vi "_Parse Session Content.vi"(11 "Text":string) -> (2 "Section":string[](array[string]), 3 "SectionContent":string[](array[string]))   [LabVIEW 2017, in "LabVIEW-Config.lvlib" / "LabVIEW-Config.lvclass"]
uses:
  LabVIEW-Config.lvclass
  LineToken.ctl
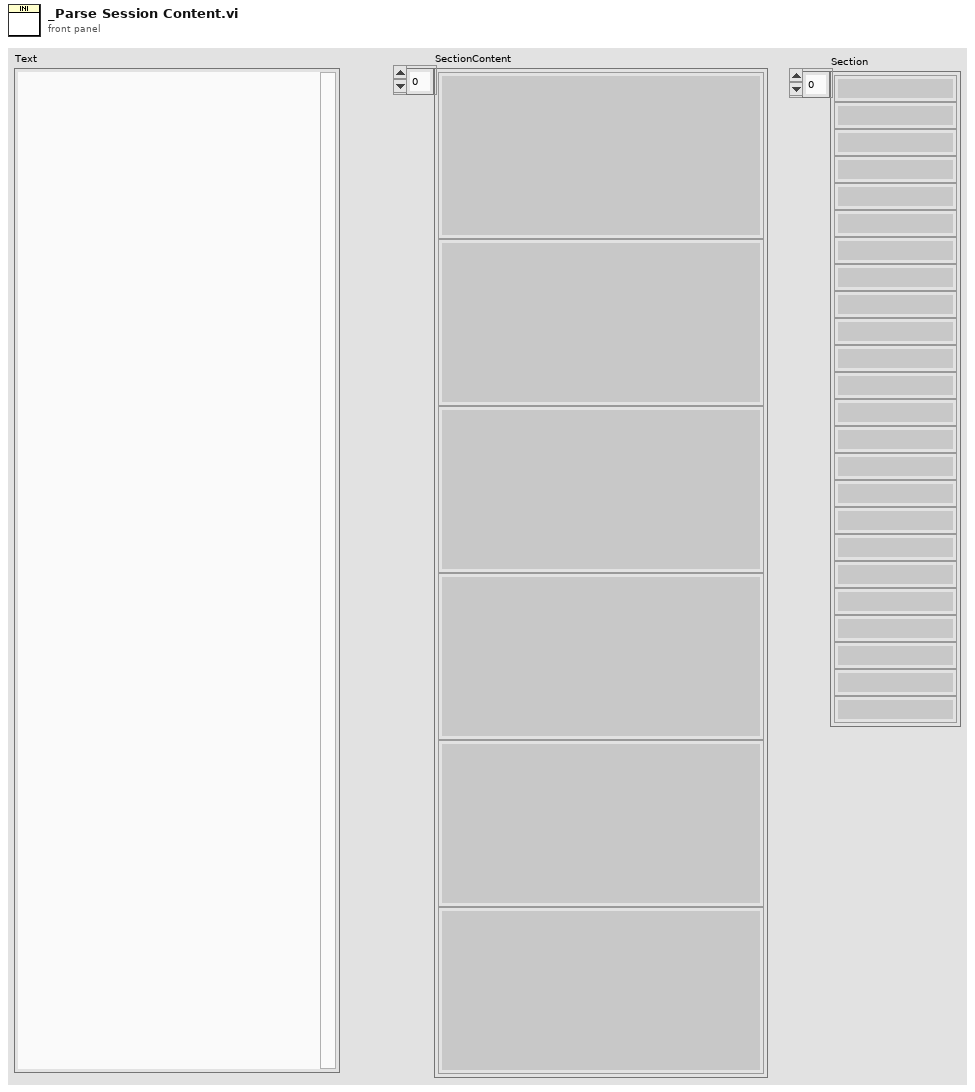
[diagram p1: front panel]
types:
  T1 = typedef "LabVIEW-Config.lvlib/LabVIEW-Config.lvclass/LineToken.ctl" = enum8{"comment", "section", "key", "more"}
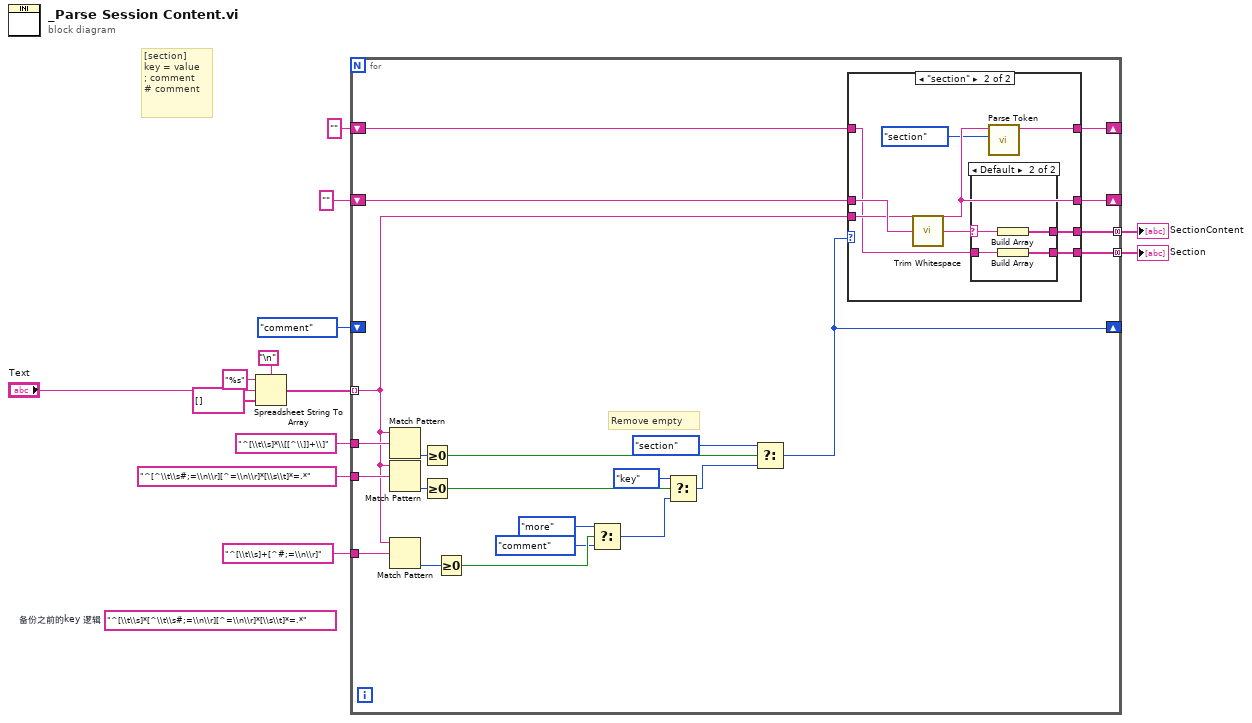
[diagram p0: block diagram]
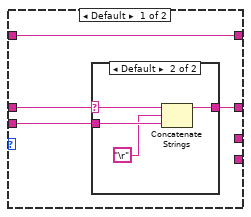
[diagram p2: hidden frame]
diagram:
  (unwired) "^[\\t\\s]*[^\\t\\s#;=\\n\\r][^=\\n\\r]*[\\s\\t]*=.*"  # 备份之前的key 逻辑
  # "[section]\nkey = value\n; comment\n# comment"
  n1 = Spreadsheet String To Array(delimiter (Tab)="\n" ("Line Feed Constant"), format string="%s", spreadsheet string="Text", array type (2D Dbl)=string[] []) -> (array=w11:string[])
  n2 = for {
    tunnel: w11 -> [w17] mode=indexing
    tunnel: "^[\\t\\s]*\\[[^\\]]+\\]" ("regular expression") -> [w36]
    tunnel: "^[^\\t\\s#;=\\n\\r][^=\\n\\r]*[\\s\\t]*=.*" ("regular expression") -> [w33]
    tunnel: "^[\\t\\s]+[^#;=\\n\\r]" ("regular expression") -> [w26]
    shift-right: [w21] -> _
    shift-left: LineToken."comment" ("Token") -> [_]
    shift-right: [w18] -> _
    shift-left: "" ("regular expression") -> [w20]
    tunnel: [w19] -> w3 mode=concatenating
    shift-right: [w16] -> _
    shift-left: "" ("Name") -> [w15]
    tunnel: [w14] -> w1 mode=concatenating
    # "Remove empty"
    n3 = Match Pattern(string=w17, regular expression=w36) -> (offset past match=w35:i32)  [unwired: 1 in, 3 out]
    n4 = Match Pattern(string=w17, regular expression=w33) -> (offset past match=w34:i32)  [unwired: 1 in, 3 out]
    n5 = Match Pattern(string=w17, regular expression=w26) -> (offset past match=w27:i32)  [unwired: 1 in, 3 out]
    n6 = Greater Or Equal To 0?(x=w35) -> (x >= 0?=w32:bool)
    n7 = Greater Or Equal To 0?(x=w34) -> (x >= 0?=w28:bool)
    n8 = Greater Or Equal To 0?(x=w27) -> (x >= 0?=w25:bool)
    n9 = Select(t=LineToken."more" ("Token"), s=w25, f=LineToken."comment" ("Token")) -> (s? t:f=w22:T1)
    n10 = Select(t=LineToken."key" ("Token"), s=w28, f=w22) -> (s? t:f=w29:T1)
    n11 = Select(t=LineToken."section" ("Token"), s=w32, f=w29) -> (s? t:f=w21:T1)
    n12 = case shown="\"section\"" w21 {
      tunnel: w20 -> [w40 w53]
      tunnel: [_ w52] -> w19
      tunnel: [w39 w50] -> w18
      tunnel: w17 -> [w38 w50]
      tunnel: [w37 w49] -> w16
      tunnel: w15 -> [w37 w47]
      tunnel: [_ w48] -> w14
      frame Default {
        n13 = case shown="Default" w40 {
          selector: w40 -> [_ w45]
          tunnel: [w41 w44] -> w39
          tunnel: w38 -> [w41 w43]
          frame "" {
          }
          frame Default {
            n14 = Concatenate Strings(w45, "\r", w43) -> (w44:string)
          }
        }
      }
      frame "section" {
        n15 = call <vilib>:"Trim Whitespace.vi"("string"=w53) -> ("trimmed string"=w51:string)  [unwired: 1 in]
        n16 = case shown="Default" w51 {
          selector: w51 -> [_ w57]
          tunnel: [_ w56] -> w52
          tunnel: [_ w54] -> w48
          tunnel: w47 -> [_ w55]
          frame "" {
          }
          frame Default {
            n17 = Build Array(w57) -> (w56:string[])
            n18 = Build Array(w55) -> (w54:string[])
          }
        }
        n19 = call "Parse Token.vi"("Token"=LineToken."section", "Line"=w50) -> ("Name"=w49:string)  [unwired: 8 in, 1 out]
      }
    }
  }
  "SectionContent" <- w3
  "Section" <- w1
